vi "PH_PILS.PC _EOLikes.vi"(0 "i ref in":refnum<vi>, 2 "serviceName":string, 3 "Value":i32, 5 "error IO":errorcluster) -> (14 "i ref out":refnum<vi>, 19 "error out":errorcluster)   [LabVIEW 2014, in "PH_PILS.lvlib"]
uses:
  PH_PILS.lvlib
  PH_Common/PH_Common.lvlib
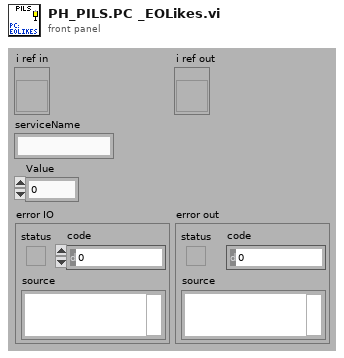
[diagram p1: front panel]
types:
  T1 = typedef "PH_PILS.lvlib/PH_PILS.i attribute.ctl" = cluster{"Boolean":cluster{"GUI Ref":refnum<vi>, "Status":i32}[], "GUI Refs Exp. Shutters":cluster{"1":refnum<vi>, "2":refnum<vi>, "3":refnum<vi>, "4":refnum<vi>}, "Tristate2Run GUI Refs":refnum<vi>[], "EO-Likes":cluster{"GUI Ref":refnum<vi>, "Status":i32}[], "Operation Mode":cluster{"Operation Mode":T2, "GUI":cluster{"Ref State":refnum<vi>, "Ref":refnum<vi>}, "Servicemode":cluster{"Tagname":string, "Status":i32}, "Labormode":cluster{"Tagname":string, "Status":i32}, "Searchmode":cluster{"Tagname":string, "Status":i32}, "Shotmode":cluster{"Tagname":string, "Status":i32}}, "Submode":cluster{"Submode":T3, "GUI":cluster{"Ref State":refnum<vi>, "Ref":refnum<vi>}, "Submode":cluster{"Tagname":string, "Status":i32}}, "Experiment":cluster{"Experiment":enum16{"unknown", "intern", "4 (Z6)", "3", "2", "1"}, "GUI":cluster{"Ref State":refnum<vi>, "Ref":refnum<vi>}, "intern":cluster{"Tagname":string, "Status":i32}, "Exp 4":cluster{"Tagname":string, "Status":i32}, "Exp 3":cluster{"Tagname":string, "Status":i32}, "Exp 2":cluster{"Tagname":string, "Status":i32}, "Exp 1":cluster{"Tagname":string, "Status":i32}}, "TristateNormal":cluster{"GUI Ref":refnum<vi>, "Status":i32}[], "Door Tags":cluster{"GUI Ref":refnum<vi>, "Status":i32}[], "GUIlessTags":cluster{"Name":string, "Status":i32}[], "Beamline GUI Refs":refnum<vi>[], "Special Boolean":cluster{"GUI Ref":refnum<vi>, "Status":i32}[], "Laserpower":cluster{"GUI Ref":refnum<vi>, "Status":i32}[], "Shutter":cluster{"GUI Ref":refnum<vi>, "Status":i32}[], "Tristate EO Like":cluster{"GUI Ref":refnum<vi>, "Status":i32}[], "PP":cluster{"GUI Ref":refnum<vi>, "Status":i32, "Head Ref":refnum<vi>, "Slider Ref":refnum<vi>}[], "Switch Knobs":cluster{"GUI Ref":refnum<vi>, "Status":i32}[], "Latch Knob GUI Refs":refnum<vi>[], "FailureCounter":i32, "Enabled Status":cluster{"Laser":i32, "PreAmp":i32, "MainAmp":i32}, "Mercury":refnum<vi>, "Instance Rods":string, "Logfile":path, "Beckhoff-Instance Internal":string, "Beckhoff-Instance External":string, "Enabling Rights":cluster{"Name":string, "Password":string, "PA?":bool, "MA?":bool, "Exp?":bool}[]}
  T2 = typedef "PH_PILS.lvlib/PH_PILS.Operation Mode.ctl" = enum16{"unknown", "Service", "Labor", "Search", "Shot"}
  T3 = typedef "PH_PILS.lvlib/PH_PILS.Submode.ctl" = enum16{"unknown", "HV-Normal", "HV-Test"}
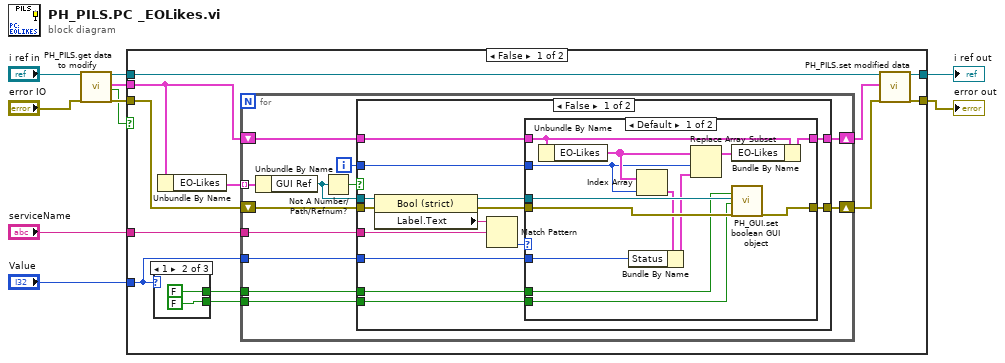
[diagram p0: block diagram]
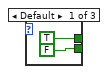
[diagram p2: hidden frame]
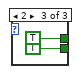
[diagram p3: hidden frame]
diagram:
  n1 = call "PH_PILS.get data to modify.vi"("i ref in"="i ref in", "error in (no error)"="error IO") -> ("i ref out"=w10:refnum<vi>, "i attribute"=w6:T1, "timed out"=w1:bool, "error out"=w8:errorcluster)  [unwired: 14 in]
  n2 = case shown="False" w1 {
    tunnel: w10 -> [w22 w73]
    tunnel: "serviceName" -> [w21 _]
    tunnel: w8 -> [w18 w72]
    tunnel: "Value" -> [w13 _]
    tunnel: w6 -> [w12 _]
    tunnel: [w16 w73] -> w3
    tunnel: [w14 w72] -> w2
    frame False {
      n3 = case shown="1" w13 {
        tunnel: [TRUE FALSE TRUE] -> w19
        tunnel: [FALSE FALSE TRUE] -> w20
        frame Default {
        }
        frame 1 {
        }
        frame 2 {
        }
      }
      n4 = Unbundle By Name(w12) -> ("EO-Likes"=w17:cluster{"GUI Ref":refnum<vi>, "Status":i32}[])
      n5 = for {
        tunnel: w17 -> [w32] mode=indexing
        tunnel: w21 -> [w40]
        shift-right: [w39] -> w15
        shift-left: w18 -> [w36]
        tunnel: w19 -> [w38]
        tunnel: w20 -> [w37]
        tunnel: w13 -> [w33]
        shift-right: [w30] -> w11
        shift-left: w12 -> [w31]
        i -> [w29]
        n6 = Unbundle By Name(w32) -> ("GUI Ref"=w34:refnum<vi>)
        n7 = Not A Number/Path/Refnum?(number/path/refnum=w34) -> (NaN/Path/Refnum?=w35:bool)
        n8 = case shown="False" w35 {
          tunnel: w40 -> [w46 _]
          tunnel: w34 -> [w52 _]
          tunnel: [w51 w71] -> w39
          tunnel: w38 -> [w50 _]
          tunnel: w37 -> [w45 _]
          tunnel: w36 -> [w49 w71]
          tunnel: w33 -> [w42 _]
          tunnel: w31 -> [w43 w70]
          tunnel: [w44 w70] -> w30
          tunnel: w29 -> [w41 _]
          frame False {
            n9 = property class="Bool (strict)"(reference=w52, error in=w49) -> (reference out=w47:refnum<vi>, error out=w48:errorcluster, "Label.Text"=w54:string)
            n10 = Match Pattern(string=w54, regular expression=w46) -> (offset past match=w53:i32)  [unwired: 1 in, 3 out]
            n11 = case shown="Default" w53 {
              tunnel: w47 -> [w67 _]
              tunnel: w48 -> [w66 w69]
              tunnel: [w65 w69] -> w51
              tunnel: w50 -> [w64 _]
              tunnel: w45 -> [w63 _]
              tunnel: w42 -> [w60 _]
              tunnel: w43 -> [w58 w68]
              tunnel: [w59 w68] -> w44
              tunnel: w41 -> [w56 _]
              frame Default {
                n12 = Unbundle By Name(w58) -> ("EO-Likes"=w57:cluster{"GUI Ref":refnum<vi>, "Status":i32}[])
                n13 = Index Array(array=w57, index=w56) -> (element=w55:cluster{"GUI Ref":refnum<vi>, "Status":i32})
                n14 = Bundle By Name(cluster=w55, "Status"=w60) -> (w61:cluster{"GUI Ref":refnum<vi>, "Status":i32})
                n15 = Replace Array Subset(array=w57, new element=w61, index=w56) -> (w62:cluster{"GUI Ref":refnum<vi>, "Status":i32}[])
                n16 = Bundle By Name(cluster=w58, "EO-Likes"=w62) -> (w59:T1)
                n17 = call "PH_GUI.set boolean GUI object.vi"("Visible (true)"=w64, "Boolean Knob GUI Ref"=w67, "Value"=w63, "error in (no error)"=w66) -> ("error out"=w65:errorcluster)  [unwired: 15 in]
              }
              frame -1 {
              }
            }
          }
          frame True {
          }
        }
      }
      n18 = call "PH_PILS.set modified data.vi"("i ref in"=w22, "i attribute"=w11, "error in (no error)"=w15) -> ("i ref out"=w16:refnum<vi>, "error out"=w14:errorcluster)  [unwired: 15 in]
    }
    frame True {
    }
  }
  "error out" <- w2
  "i ref out" <- w3
